vi "U8toFXP.vi"(1 "Input":u8, 2 "Values memory":refnum<k21>) -> (0 "Output":fxp<+/-,48,16>)   [LabVIEW 2018]
uses:
  <vilib>/Utility/error.llb/Clear Errors.vi
  <vilib>/rvi/Emulation/niFpgaSctlEmulationGetInTimedLoop.vi
  <vilib>/rvi/DataTransferAndStorage/Container/Common/niFpgaContainerGetUniqueNameForEmu.vi
  <vilib>/rvi/DataTransferAndStorage/Container/Common/niFpgaContainerSetEmuInfo.vi
  <vilib>/rvi/eio/common/nirviEmuReportErrorAndStop.vi
  <vilib>/rvi/DataTransferAndStorage/Container/Common/niFpgaContainerExecOnDevCompGetState.vi
  <vilib>/rvi/Emulation/niFpgaEmulationIsFPGAContextNoSignature.vi
  <vilib>/rvi/Memory/Memory_Emulation/niFpgaMemoryEmulationCacheClearOnFirstRun.vi
  <vilib>/rvi/Memory/Memory_Emulation/nirvimemoryEmulationManagerCache_MakeExclusive.vi
  <vilib>/rvi/Memory/Memory_Emulation/niFpgaMemoryEmulationValidateCache.vi
  <vilib>/rvi/Memory/Memory_Emulation/nirvimemoryEmulationManagerCache_InsertValue.vi
  <vilib>/rvi/Memory/Memory_Emulation/nirvimemoryEmulationManagerCache_ReleaseExclusive.vi
  <vilib>/rvi/Memory/Memory_Emulation/nirvimemoryEmulationManagerCache_GetValue.vi
  <vilib>/rvi/Memory/Memory_Emulation/nirvimemoryEmulationManagerCache_SetValue.vi
  <vilib>/rvi/Emulation/niFpgaProcessEmulError.vi
  <vilib>/rvi/errors/nirviReportUnexpectedCaseInternalError (U32).vi
  <vilib>/rvi/Emulation/niFpgaSctlEmulationResourceMgr.vi
  <vilib>/rvi/LocalResourceManager/LocalResourceManager.xnode
  <vilib>/rvi/DataTransferAndStorage/Container/XNode/niFpgaContainer.xnode
  <vilib>/rvi/DataTransferAndStorage/Register/Emulation/niFpgaRegisterEmulationRefIn.vi
  <vilib>/rvi/Memory/Memory_Emulation/niFpgaMemoryEmulationRefIn.vi
panel:
  # "Stores state information in registers\nConverts C<addres>=value,C<a.. data into memory entrie"
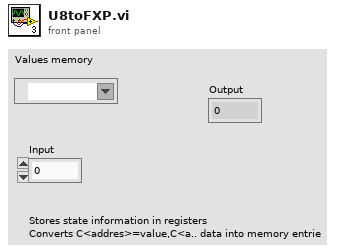
[diagram p1: front panel]
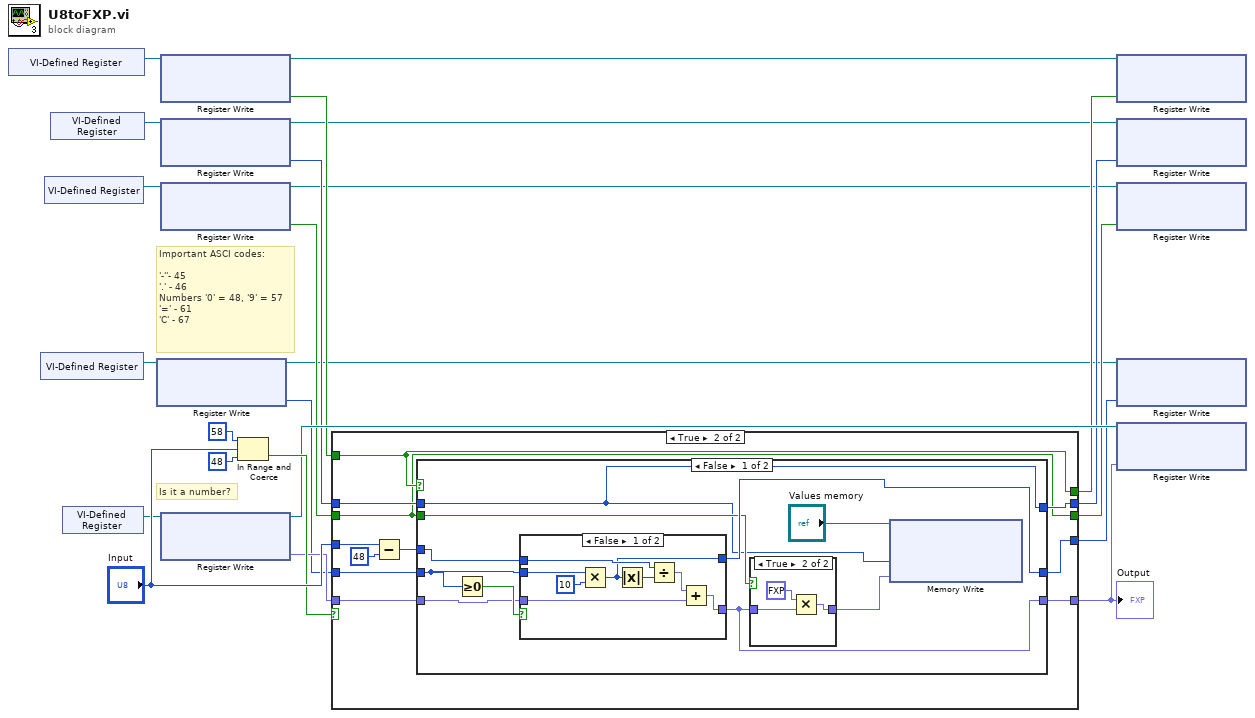
[diagram p0: block diagram]
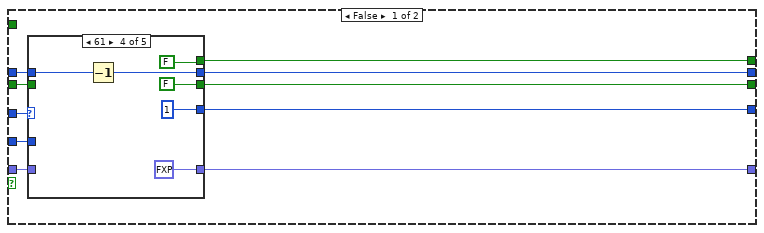
[diagram p2: hidden frame]
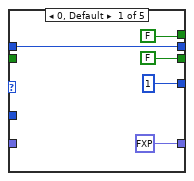
[diagram p3: hidden frame]
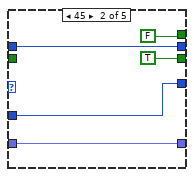
[diagram p4: hidden frame]
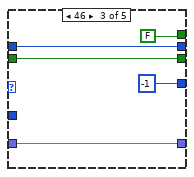
[diagram p5: hidden frame]
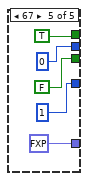
[diagram p6: hidden frame]
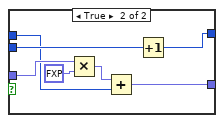
[diagram p8: hidden frame]
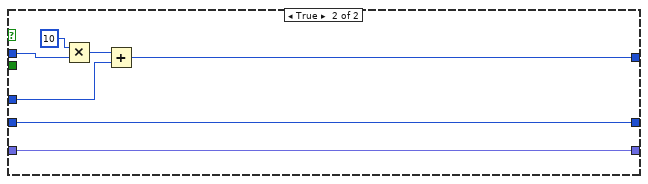
[diagram p9: hidden frame]
diagram:
  # "Is it a number?"
  # "Important ASCI codes:\n\n'-''- 45\n'.' - 46\nNumbers '0' = 48, '9' = 57\n'=' - 61\n'C' - 67"
  n1 = xnode "VI-Defined Register"() -> ("Register Out"=w15:refnum<k21>)
  n2 = xnode "VI-Defined Register"() -> ("Register Out"=w3:refnum<k21>)
  n3 = xnode "VI-Defined Register"() -> ("Register Out"=w7:refnum<k21>)
  n4 = xnode "VI-Defined Register"() -> ("Register Out"=w11:refnum<k21>)
  n5 = xnode "VI-Defined Register"() -> ("Register Out"=w20:refnum<k21>)
  n6 = xnode "Register Write"("Register In"=w3) -> ("Data"=w1:i16, "Register Out"=w2:refnum<k21>)
  n7 = xnode "Register Write"("Register In"=w15) -> ("Data"=w13:bool, "Register Out"=w14:refnum<k21>)
  n8 = xnode "Register Write"("Register In"=w11) -> ("Data"=w9:u8, "Register Out"=w10:refnum<k21>)
  n9 = xnode "Register Write"("Register In"=w7) -> ("Data"=w5:bool, "Register Out"=w6:refnum<k21>)
  n10 = xnode "Register Write"("Register In"=w20) -> ("Data"=w19:fxp<+/-,24,8>, "Register Out"=w18:refnum<k21>)
  n11 = In Range and Coerce(upper limit=u8 58, x="Input", lower limit=u8 48) -> (In Range?=w21:bool)  [unwired: 1 out]
  n12 = case shown="True" w21 {
    tunnel: "Input" -> [w34 w70]
    tunnel: [w32 w68] -> w17
    tunnel: w19 -> [w31 w67]
    tunnel: [w33 w66] -> w4
    tunnel: w1 -> [w28 w65]
    tunnel: [w30 w61] -> w8
    tunnel: w5 -> [w29 w61]
    tunnel: w9 -> [w27 w63]
    tunnel: [w26 w62] -> w12
    tunnel: w13 -> [_ w64]
    tunnel: [w25 w64] -> w16
    frame False {
      n13 = case shown="61" w34 {
        tunnel: [1 w44 -1 1 ("Data") 1 ("Data")] -> w33
        tunnel: [fxp<+/-,24,8> 0.0 ("Data") w42 w48 fxp<+/-,24,8> 0.0 ("Data") fxp<+/-,24,8> 0.0 ("Data")] -> w32
        tunnel: w31 -> [_ w42 w48 _ _]
        tunnel: [FALSE ("Data") TRUE ("Data") w47 FALSE ("Data") FALSE ("Data")] -> w30
        tunnel: w29 -> [_ _ w47 _ _]
        tunnel: w28 -> [_ w44 _ _ _]
        tunnel: w27 -> [w36 w41 w46 w54 _]
        tunnel: [w36 w41 w46 w50 u8 0 ("Data")] -> w26
        tunnel: [FALSE ("Data") FALSE ("Data") FALSE ("Data") FALSE ("Data") TRUE ("Data")] -> w25
        frame 0, Default {
        }
        frame 45 {
        }
        frame 46 {
        }
        frame 61 {
          n14 = Decrement(x=w54) -> (x-1=w50:u8)
        }
        frame 67 {
        }
      }
    }
    frame True {
      n15 = Subtract(x=w70, y=u8 48) -> (x-y=w69:u8)
      n16 = case shown="False" w64 {
        tunnel: w69 -> [w80 w104]
        tunnel: [w75 w101] -> w68
        tunnel: w67 -> [w79 w101]
        tunnel: [w78 w102] -> w66
        tunnel: w65 -> [w77 w102]
        tunnel: w63 -> [w73 w106]
        tunnel: [w73 w103] -> w62
        tunnel: w61 -> [w76 _]
        frame False {
          n17 = Greater Or Equal To 0?(x=w77) -> (x >= 0?=w81:bool)
          n18 = case shown="False" w81 {
            tunnel: w79 -> [w90 w100]
            tunnel: [w87 w98] -> w78
            tunnel: [w86 w95] -> w75
            tunnel: w80 -> [w93 w94]
            tunnel: w77 -> [w88 w97]
            frame False {
              n19 = Multiply(x=w88, y=10) -> (x*y=w87:i32)
              n20 = Absolute Value(x=w87) -> (abs(x)=w92:i32)
              n21 = Divide(x=w93, y=w92) -> (x/y=w89:fxp<+/-,24,8>)
              n22 = Add(x=w89, y=w90) -> (x+y=w86:fxp<+/-,24,8>)
            }
            frame True {
              n23 = Multiply(x=w100, y=fxp<+/-,24,8> 10.0) -> (x*y=w99:fxp<+/-,48,16>)
              n24 = Add(x=w99, y=w94) -> (x+y=w95:fxp<+/-,48,16>)
              n25 = Increment(x=w97) -> (x+1=w98:i16)
            }
          }
          n26 = case shown="True" w76 {
            tunnel: [w82 w84] -> w72
            tunnel: w75 -> [w82 w85]
            frame False {
            }
            frame True {
              n27 = Multiply(x=fxp<+/-,48,16> -1.0, y=w85) -> (x*y=w84:fxp<+/-,64,30>)
            }
          }
          n28 = xnode "Memory Write"("Address"=w73, "Data"=w72, "Memory In"="Values memory") -> ()  [unwired: 1 out]
        }
        frame True {
          n29 = Multiply(x=u8 10, y=w106) -> (x*y=w105:u8)
          n30 = Add(x=w105, y=w104) -> (x+y=w103:u8)
        }
      }
    }
  }
  "Output" <- w17
  n31 = xnode "Register Write"("Data"=w16, "Register In"=w14) -> ()  [unwired: 1 out]
  n32 = xnode "Register Write"("Data"=w12, "Register In"=w10) -> ()  [unwired: 1 out]
  n33 = xnode "Register Write"("Data"=w8, "Register In"=w6) -> ()  [unwired: 1 out]
  n34 = xnode "Register Write"("Data"=w4, "Register In"=w2) -> ()  [unwired: 1 out]
  n35 = xnode "Register Write"("Data"=w17, "Register In"=w18) -> ()  [unwired: 1 out]
